vi "upload_data.vi"(8 "error in (no error)":errorcluster, 11 "ExperimentVariables in":refnum<class "ExperimentVariables.lvclass">) -> (0 "error out":errorcluster, 3 "ExperimentVariables out":refnum<class "ExperimentVariables.lvclass">)   [LabVIEW 2012, in "ExperimentVariables.lvclass"]
uses:
  ExperimentVariables.lvclass
  ExperimentVariables.lvclass/ExperimentVariables.ctl
panel:
  out "new path":path
  out "date":string
  out "time":string
  out "no time or date path":path
  out "network date and time path":path
  out "network date path":path
  out "Variable Settings.Network Data Path":path
  out "no time path":path
  out "timestamped data path":path
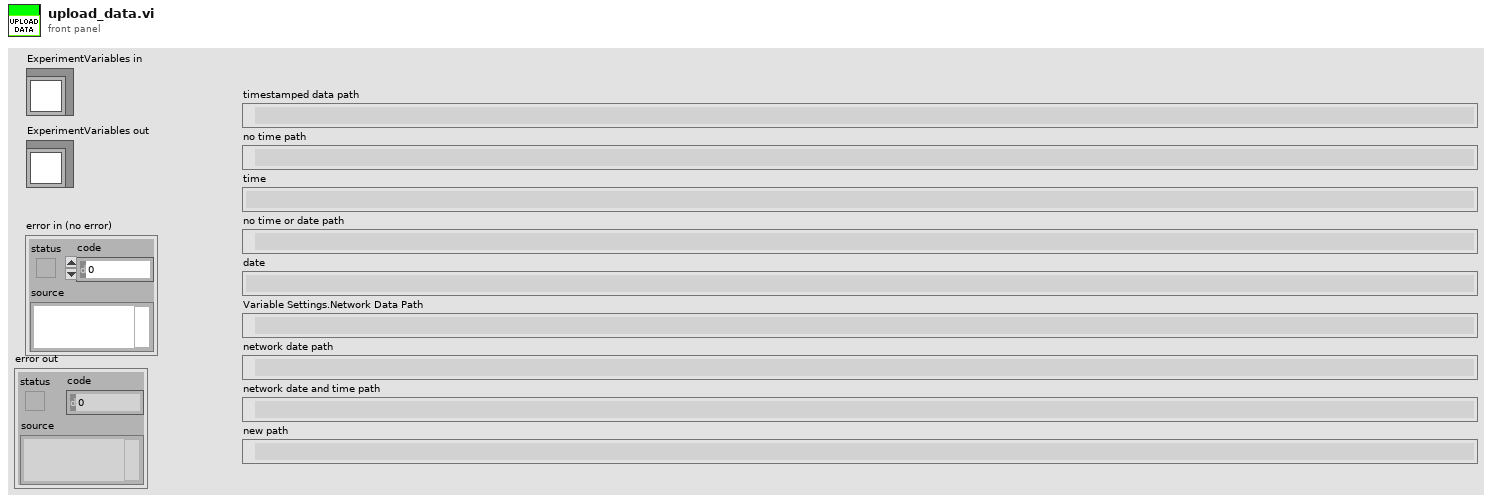
[diagram p1: front panel]
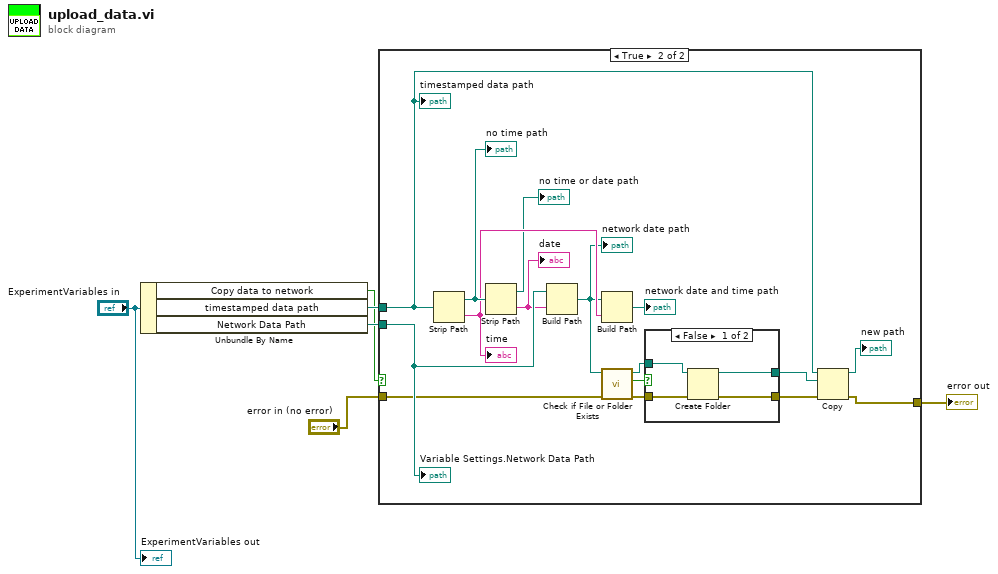
[diagram p0: block diagram]
diagram:
  n1 = Unbundle By Name("ExperimentVariables in") -> ("Copy data to network"=w3:bool, "timestamped data path"=w5:path, "Network Data Path"=w4:path)
  n2 = case shown="True" w3 {
    tunnel: w5 -> [_ w23]
    tunnel: w4 -> [_ w21]
    tunnel: "error in (no error)" -> [w7 w9]
    tunnel: [w7 w8] -> w1
    frame False {
    }
    frame True {
      n3 = Strip Path(path=w23) -> (stripped path=w22:path, name=w19:string)
      "no time path" <- w22
      "time" <- w19
      n4 = Strip Path(path=w22) -> (stripped path=→"no time or date path":path, name=w20:string)
      "date" <- w20
      n5 = Build Path(base path=w21, name or relative path=w20) -> (appended path=w11:path)
      "network date path" <- w11
      n6 = Build Path(base path=w11, name or relative path=w19) -> (appended path=→"network date and time path":path)
      n7 = call <vilib>:"Check if File or Folder Exists.vi"("error in (no error)"=w9, "path"=w11) -> ("error out"=w14:errorcluster, "file or folder exists?"=w15:bool, "dup path"=w10:path)  [unwired: 7 in]
      n8 = case shown="False" w15 {
        tunnel: w14 -> [w27 w29]
        tunnel: [w26 w29] -> w13
        tunnel: w10 -> [w25 w28]
        tunnel: [w24 w28] -> w12
        frame False {
          n9 = Create Folder(path (use dialog)=w25, error in=w27) -> (created path=w24:path, error out=w26:errorcluster)  [unwired: 1 in, 1 out]
        }
        frame True {
        }
      }
      n10 = Copy(8:w13, 10:w12, 11:w23) -> (0:w8:errorcluster, 3:→"new path":path)  [unwired: 2 in, 1 out]
      "timestamped data path" <- w23
      "Variable Settings.Network Data Path" <- w21
    }
  }
  "error out" <- w1
  "ExperimentVariables out" <- "ExperimentVariables in"
